vi "Read Spreadsheet Settings all.vi"() -> (3 "Autonomous Data":T1(array[cluster]))   [LabVIEW 2017]
uses:
  <vilib>/Utility/file.llb/Read Delimited Spreadsheet (string).vi
panel:
  out "error out":errorcluster
  out "all rows":string[][](array[string])
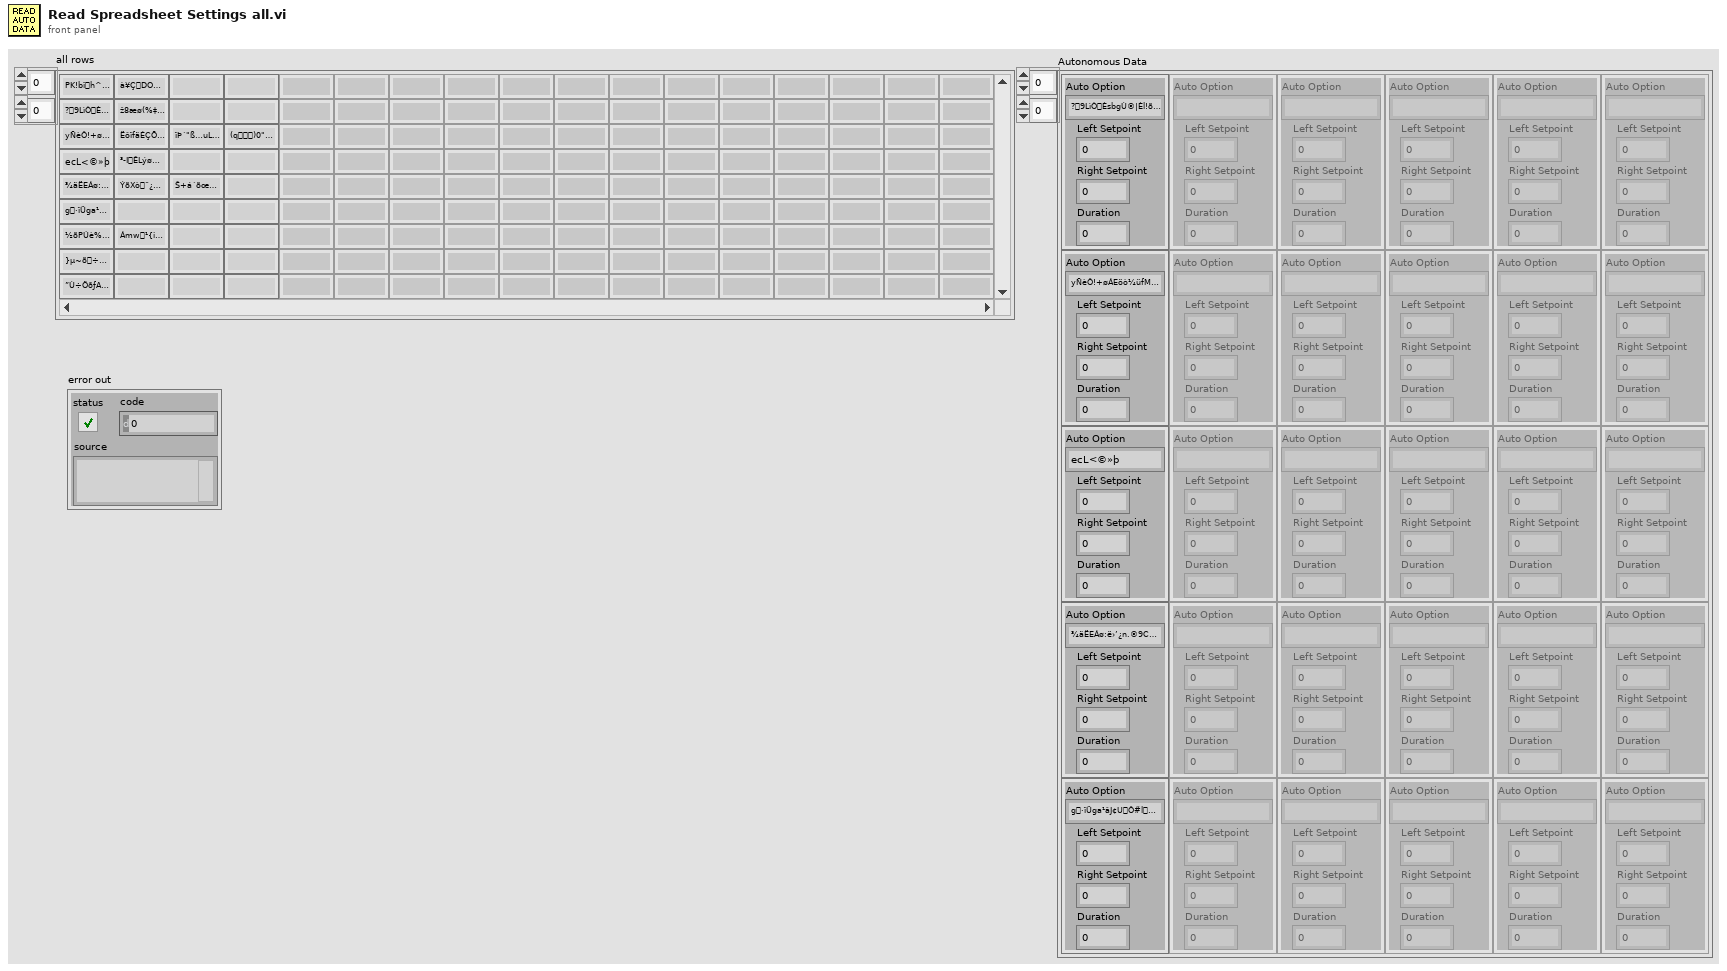
[diagram p1: front panel]
types:
  T1 = cluster{"Auto Option":string, "Left Setpoint":dbl, "Right Setpoint":dbl, "Duration":dbl}[][]
  T2 = cluster{"Auto Option":string, "Left Setpoint":dbl, "Right Setpoint":dbl, "Duration":dbl}
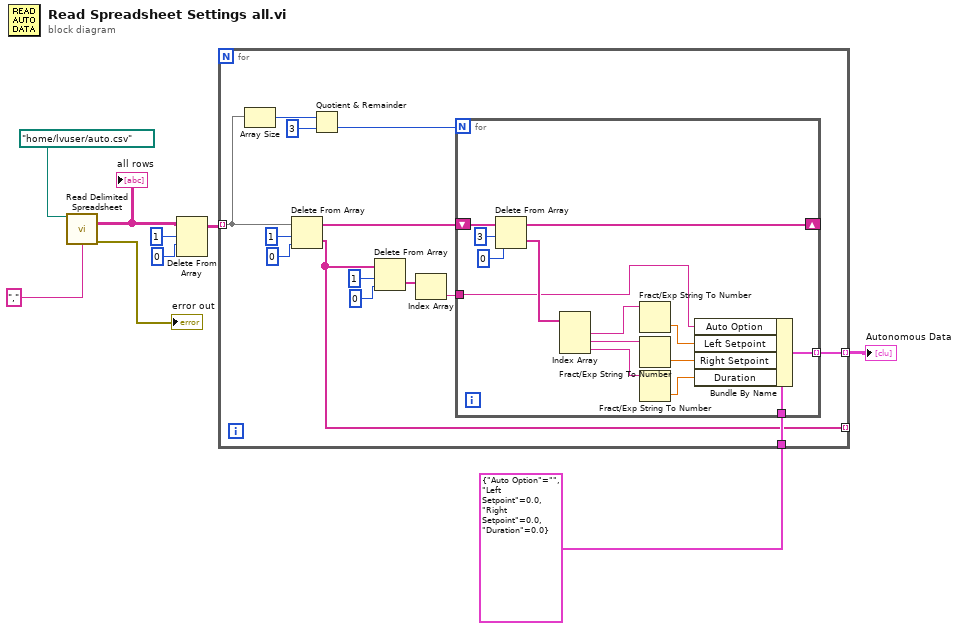
[diagram p0: block diagram]
diagram:
  n1 = call-poly <vilib>:"Read Delimited Spreadsheet.vi"("file path (dialog if empty)"=path "/home/lvuser/auto.csv" ("Filepath"), "delimiter (\\t)"="," ("delimiter (\\t)")) -> ("all rows"=w4:string[][], "error out"=→"error out":errorcluster)  [unwired: 8 in, 4 out]
  "all rows" <- w4
  n2 = Delete From Array(array=w4, length=1, index (row)=0 ("index")) -> (array with subset deleted=w3:string[][])  [unwired: 1 in, 1 out]
  n3 = for {
    tunnel: w3 -> [w18] mode=indexing
    tunnel: T2 {"Auto Option"="", "Left Setpoint"=0.0, "Right Setpoint"=0.0, "Duration"=0.0} -> [w16]
    tunnel: [w15] -> w2 mode=indexing
    tunnel: [w13] -> _ mode=indexing
    n4 = Array Size(array=w18) -> (size(s)=w23:i32)
    n5 = Delete From Array(array=w18, length=1, index=0) -> (deleted portion=w13:string[], array with subset deleted=w17:string[])
    n6 = Quotient & Remainder(x=w23, y=3) -> (floor(x/y)=w21:i32)  [unwired: 1 out]
    n7 = Delete From Array(array=w13, length=1, index=0) -> (deleted portion=w10:string[])  [unwired: 1 out]
    n8 = Index Array(array=w10) -> (element=w11:string)  [unwired: 1 in]
    n9 = for {
      N: w21 -> [_]
      shift-right: [w36] -> _
      shift-left: w17 -> [w37]
      tunnel: w16 -> [w33]
      tunnel: [w25] -> w15 mode=indexing
      tunnel: w11 -> [w24]
      n10 = Delete From Array(array=w37, length=3, index=0) -> (deleted portion=w32:string[], array with subset deleted=w36:string[])
      n11 = Index Array(array=w32) -> (element #1=w31:string, element #2=w30:string, element #3=w29:string)  [unwired: 3 in]
      n12 = Fract/Exp String To Number(string=w31) -> (number=w28:dbl)  [unwired: 3 in, 1 out]
      n13 = Fract/Exp String To Number(string=w30) -> (number=w27:dbl)  [unwired: 3 in, 1 out]
      n14 = Fract/Exp String To Number(string=w29) -> (number=w26:dbl)  [unwired: 3 in, 1 out]
      n15 = Bundle By Name(cluster=w33, "Auto Option"=w24, "Left Setpoint"=w28, "Right Setpoint"=w27, "Duration"=w26) -> (w25:T2)
    }
  }
  "Autonomous Data" <- w2
